vi "Actor Core.vi"(8 "error in":errorcluster, 11 "Sim Compass in":refnum<class "Sim Compass.lvclass">) -> (0 "error out":errorcluster, 3 "Actor out":refnum<class "Actor.lvclass">)   [LabVIEW 2015, in "Sim Compass.lvlib" / "Sim Compass.lvclass"]
doc: "(<B>Filename</B>: Actor Framework.lvlib:Actor.lvclass:Actor Core.vi)\n\nReceives messages to the actor, reacts to them, and initiates any error handling that may shut the actor down.\n\nDescendant classes may override this VI to append parallel tasks for the actor to complete while it handles messages. Overrides use the Call Parent Method node."
uses:
  Sim Compass.lvclass
  <vilib>/ActorFramework/Actor/Actor.lvclass
  Libraries/RDS Instruments/Compass/Compass Data.ctl
  <vilib>/ActorFramework/Actor/Actor.lvclass/Actor.ctl
  <vilib>/ActorFramework/Message Enqueuer/Message Enqueuer.lvclass/Message Enqueuer.ctl
  Libraries/RDS Child Messages/Compass/Compass Data Message.lvclass
  Libraries/RDS Framework/RDS Message ID.ctl
  Libraries/RDS Framework/RDS Message Class/RDS Message.lvclass/RDS Message.ctl
  Libraries/RDS Child Messages/Compass/Compass Data Message.lvclass/Compass Data Message.ctl
  <vilib>/ActorFramework/Message Enqueuer/Init from Existing Queue.vi
  <vilib>/ActorFramework/Message Enqueuer/Message Enqueuer.lvclass
  RDS Parent Actor/RDS Parent Actor/RDS Parent Actor.lvclass
  Libraries/RDS Framework/RDS Message Class/RDS Message.lvclass
  Libraries/RDS Child Messages/RDS Child Messages.lvlib
  Libraries/RDS Instruments/RDS Instrument Library.lvlib
panel:
  in  "OK Button":bool
  in  "Compass Data":T1
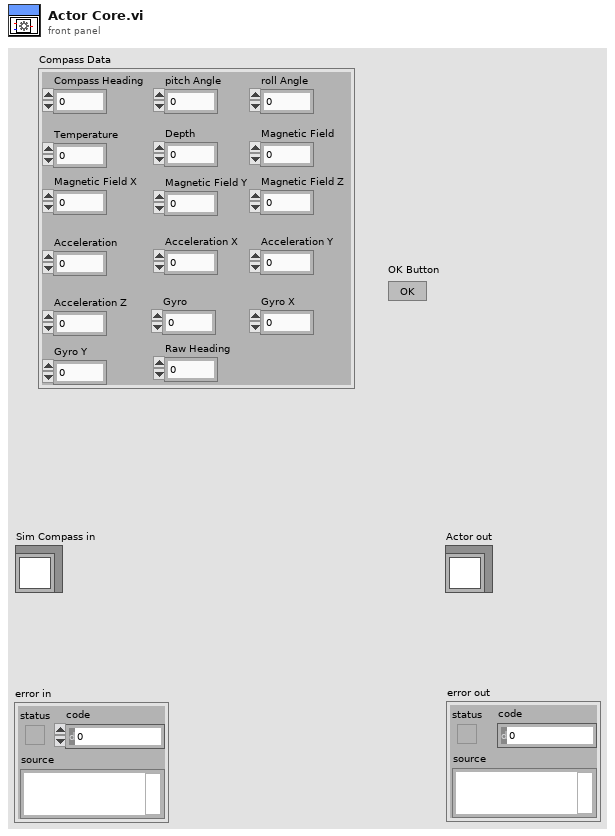
[diagram p1: front panel]
types:
  T1 = typedef "RDS Instrument Library.lvlib/Compass Data.ctl" = cluster{"Compass Heading":sgl, "pitch Angle":sgl, "roll Angle":sgl, "Temperature":sgl, "Depth":sgl, "Magnetic Field":sgl, "Magnetic Field X":sgl, "Magnetic Field Y":sgl, "Magnetic Field Z":sgl, "Acceleration":sgl, "Acceleration X":sgl, "Acceleration Y":sgl, "Gyro":sgl, "Gyro X":sgl, "Acceleration Z":sgl, "Gyro Y":sgl, "Raw Heading":sgl}
  T2 = typedef "RDS Child Messages.lvlib/RDS Message ID.ctl" = enum16{"RDS Hello World", "String Message", "AIP_Status", "AIP_Command", "GPS_Data", "MCB_Command", "MCB_Status", "Compass_Data", "Depth_Data", "Battery_Data", "Contoller_State", "Set_Mag_Dev", "BTB_Shutdown", "State_Sample_Request", "State_Sample", "PID_Gains_Set", "Helm_Limiter_Set", "Helm_Heading_Command", "Helm_Steering_Command", "Helm_Status", "Controller_Message", "AIP_Set_Min_Depth", "Mission_Controller_State", "Mission_Upload", "Mission_Set_Op_and_Run", "Mission_Settings_Set"}
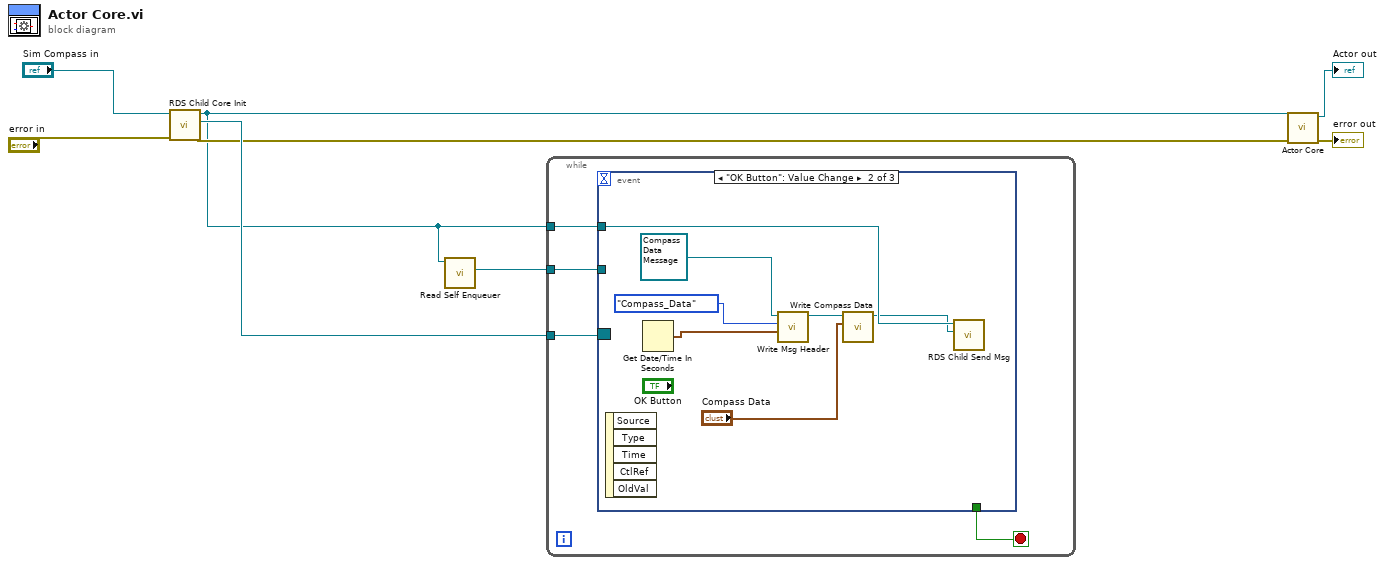
[diagram p0: block diagram]
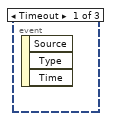
[diagram p2: hidden frame]
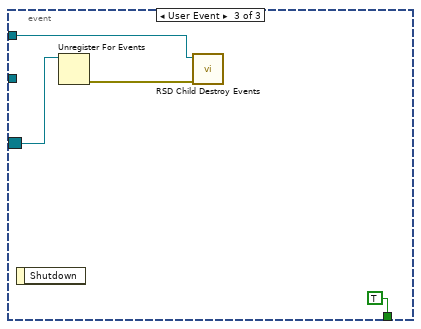
[diagram p3: hidden frame]
diagram:
  n1 = call "RDS Child Core Init.vi"("error in (no error)"="error in", "RDS Parent Actor in"="Sim Compass in") -> ("error out"=w4:errorcluster, "Event Registration Refnum"=w6:refnum<event-registration>, "RDS Parent Actor out"=w1:refnum<class "Sim Compass.lvclass">)  [unwired: 6 in, 1 out]
  n2 = call <vilib>:"Read Self Enqueuer.vi"("Actor"=w1) -> ("Self Enqueuer"=w5:refnum<class "Message Enqueuer.lvclass">)  [unwired: 10 in]
  n3 = while {
    tunnel: w6 -> [w11]
    tunnel: w1 -> [w12]
    tunnel: w5 -> [w9]
    stop <- w10 stop-if-true
    n4 = event shown="[1] \"OK Button\": Value Change" {
      selector: w11 -> [_ _ w21]
      dyn-events: _ -> [_ _ _]
      timeout: _ -> [_ _ _]
      tunnel: w12 -> [_ w14 w20]
      tunnel: [_ _ TRUE] -> w10
      tunnel: w9 -> [_ _ _]
      event Timeout {
        n5 = event-data() -> ()  [unwired: 1 in, 3 out]
      }
      event "OK Button": Value Change {
        n6 = event-data() -> ()  [unwired: 1 in, 5 out]
        n7 = Get Date/Time In Seconds() -> (seconds since 1Jan1904=w18:timestamp)
        n8 = call "Write Msg Header.vi"("Time Stamp"=w18, "Msg ID"=RDS_Message_ID."Compass_Data", "RDS Message in"=refnum<class "Compass Data Message.lvclass"> refnum ("RDS Child Messages.lvlib:Compass Data Message.lvclass")) -> ("RDS Message out"=w16:refnum<class "Compass Data Message.lvclass">)  [unwired: 7 in, 1 out]
        n9 = call "Write Compass Data.vi"("Compass Data"="Compass Data", "Compass Data Message in"=w16) -> ("Compass Data Message out"=w13:refnum<class "Compass Data Message.lvclass">)  [unwired: 8 in, 1 out]
        n10 = call "RDS Child Send Msg.vi"("RDS Message"=w13, "RDS Parent Actor in"=w14) -> ()  [unwired: 8 in, 2 out]
      }
      event User Event {
        n11 = event-data() -> ()  [unwired: 1 in, 1 out]
        n12 = Unregister For Events(event registration refnum=w21) -> (error out=w22:errorcluster)  [unwired: 1 in]
        n13 = call "RSD Child Destroy Events.vi"("error in (no error)"=w22, "RDS Parent Actor in"=w20) -> ()  [unwired: 8 in, 2 out]
      }
    }
  }
  n14 = call-parent "Actor Core.vi"("error in"=w4, "Actor in"=w1) -> ("error out"=→"error out":errorcluster, "Actor out"=→"Actor out":refnum<class "Actor.lvclass">)  [unwired: 8 in]
